vi "Multichannel_Division.vi"(9 "Array in":u64[](array[numeric])) -> (0 "Array Out1":dbl[](array[numeric]), 3 "Array Out0":dbl[](array[numeric]))   [LabVIEW 2016]
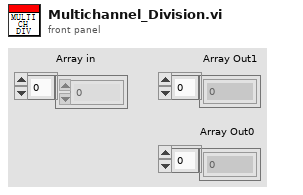
[diagram p1: front panel]
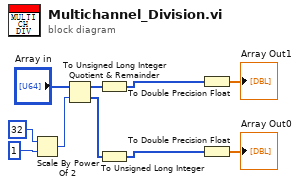
[diagram p0: block diagram]
diagram:
  n1 = Scale By Power Of 2(n=i16 32, x=u64 1) -> (x*2^n=w10:u64)
  n2 = Quotient & Remainder(x="Array in", y=w10) -> (x-y*floor(x/y)=w9:u64[], floor(x/y)=w8:u64[])
  n3 = To Unsigned Long Integer(number=w9) -> (unsigned 32bit integer=w4:u32[])
  n4 = To Unsigned Long Integer(number=w8) -> (unsigned 32bit integer=w3:u32[])
  n5 = To Double Precision Float(number=w4) -> (double precision float=→"Array Out1":dbl[])
  n6 = To Double Precision Float(number=w3) -> (double precision float=→"Array Out0":dbl[])
